vi "Array Parser.vi"() -> (1 "Auto Routines":string[](array[string]), 2 "List of Files":string[](array[string]), 3 "CSV Data":string[][][](array[string]))   [LabVIEW 2016]
uses:
  <vilib>/Utility/sysdir.llb/System Directory Type.ctl
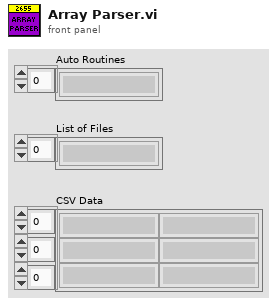
[diagram p1: front panel]
types:
  T1 = typedef "System Directory Type.ctl" = i32
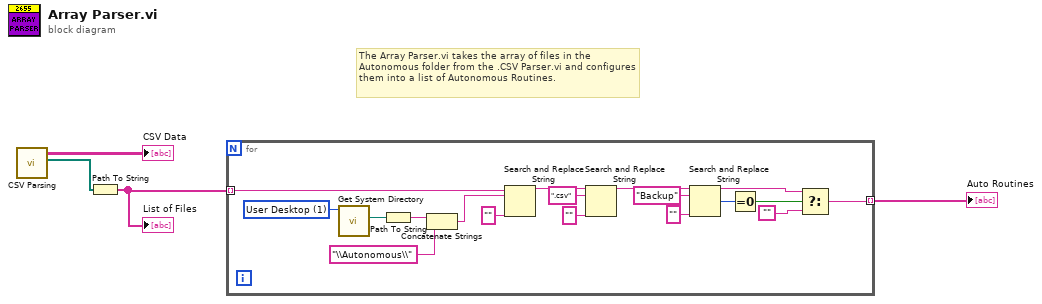
[diagram p0: block diagram]
diagram:
  # "The Array Parser.vi takes the array of files in the Autonomous folder from the .CSV Parser.vi and configures them into a list of Autonomous Routines."
  n1 = call "CSV Parsing.vi"() -> ("Files in Directory"=w4:path[], "CSV Data"=→"CSV Data":string[][][])  [unwired: 10 in]
  n2 = Path To String(path=w4) -> (string=w3:string[])
  "List of Files" <- w3
  n3 = for {
    tunnel: w3 -> [w13] mode=indexing
    tunnel: [w9] -> w2 mode=indexing
    w18 = T1 1 items=["User Home"=0, "User Desktop"=1, "User Documents"=2, "User Application Data"=3, "User Preferences"=4, "User Temporary"=5, "Public Documents"=6, "Public Application Data"=7, "Public Preferences"=8, "Public Cache"=13, "System Core Libraries"=9, "System Installed Libraries"=10, "Application Files"=11, "Boot Volume Root"=12] ("system directory type")
    n4 = call <vilib>:"Get System Directory.vi"("system directory type"=w18) -> ("system directory"=w17:path)  [unwired: 10 in]
    n5 = Path To String(path=w17) -> (string=w16:string)
    n6 = Concatenate Strings(w16, "\\Autonomous\\" ("string")) -> (w14:string)
    n7 = Search and Replace String(input string=w13, search string=w14, replace string="" ("replace string (\"\")")) -> (result string=w19:string)  [unwired: 5 in, 3 out]
    n8 = Search and Replace String(input string=w19, search string=".csv", replace string="" ("replace string (\"\")")) -> (result string=w11:string)  [unwired: 5 in, 3 out]
    n9 = Search and Replace String(input string=w11, search string="Backup", replace string="" ("replace string (\"\")")) -> (result string=w10:string, number of replacements=w7:i32)  [unwired: 5 in, 2 out]
    n10 = Equal To 0?(x=w7) -> (x = 0?=w6:bool)
    n11 = Select(t=w10, s=w6, f="") -> (s? t:f=w9:string)
  }
  "Auto Routines" <- w2
